vi "load channel file.vi"(8 "error in":errorcluster, 10 "Group Names":string[](array[string]), 11 "Channel List":path) -> (0 "error out":errorcluster, 1 "ACTIVE":T3 {"Channels in Group"."Card.Channel" format="%.2f"}, 2 "GROUP00":T3 {"Channels in Group"."Card.Channel" format="%.2f"}, 3 "Groups":T4(array[cluster]) {"Channels in Group"."Card.Channel" format="%.2f"}, 5 "Array":T1[](array[typedef]) {"Vfile (V)" format="%.1f V"; "Vswmax (V)" format="%#_g V"; "Iset (A)" format="%.2pA"; "Imon (A)" format="%.2pA"; "Vset (V)" format="%#_g V"; "Vmon (V)" format="%.1f V"})   [LabVIEW 2018]
uses:
  channel.ctl
  channel_cluster.ctl
  <vilib>/Utility/file.llb/Read Delimited Spreadsheet (string).vi
  string to bool small.vi
  fr string to dbl small.vi
  dec string to i32 small.vi
  CAEN globals.vi
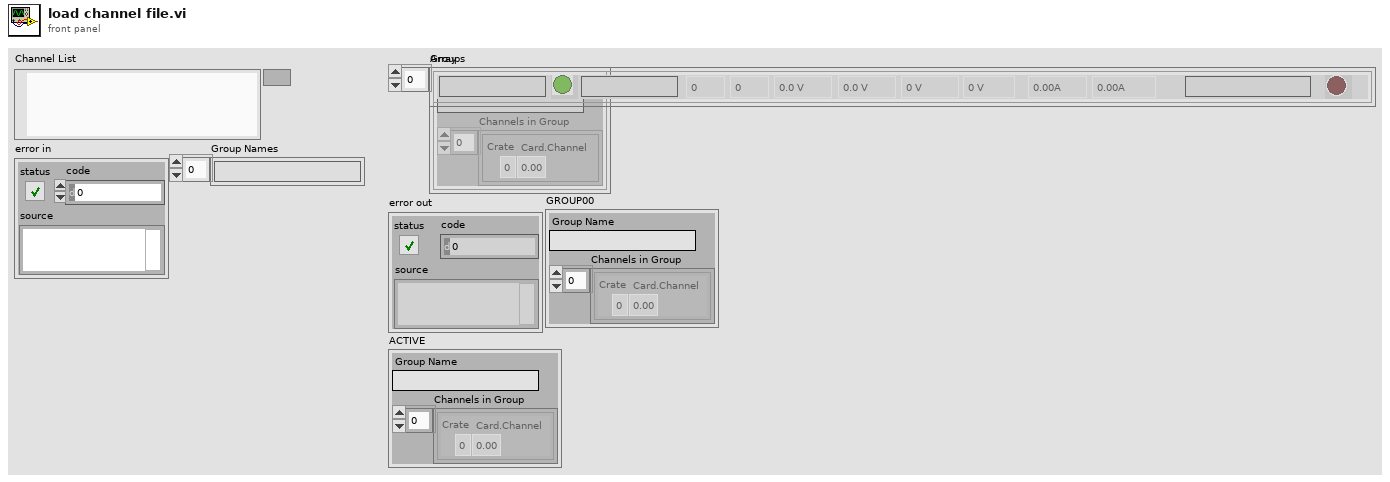
[diagram p1: front panel]
types:
  T1 = typedef "channel_cluster.ctl" = cluster{"Channel Name":string, "Crate":i32, "Card Type":string, "Card":i32, "Channel":i32, "Status Icon":picture, "Vmon (V)":dbl, "Vset (V)":dbl, "Imon (A)":dbl, "Iset (A)":dbl, "Timestamp":string, "ON/OFF":bool, "Status":string, "Vswmax (V)":dbl, "Flag":bool, "Vfile (V)":dbl, "Error Logged":bool[], "enable_file":bool}
  T2 = typedef "channel.ctl" = cluster{" Card.Channel":dbl, "Crate":i32}
  T3 = cluster{"Group Name":string, "Channels in Group":T2[]}
  T4 = cluster{"Group Name":string, "Channels in Group":T2[]}[]
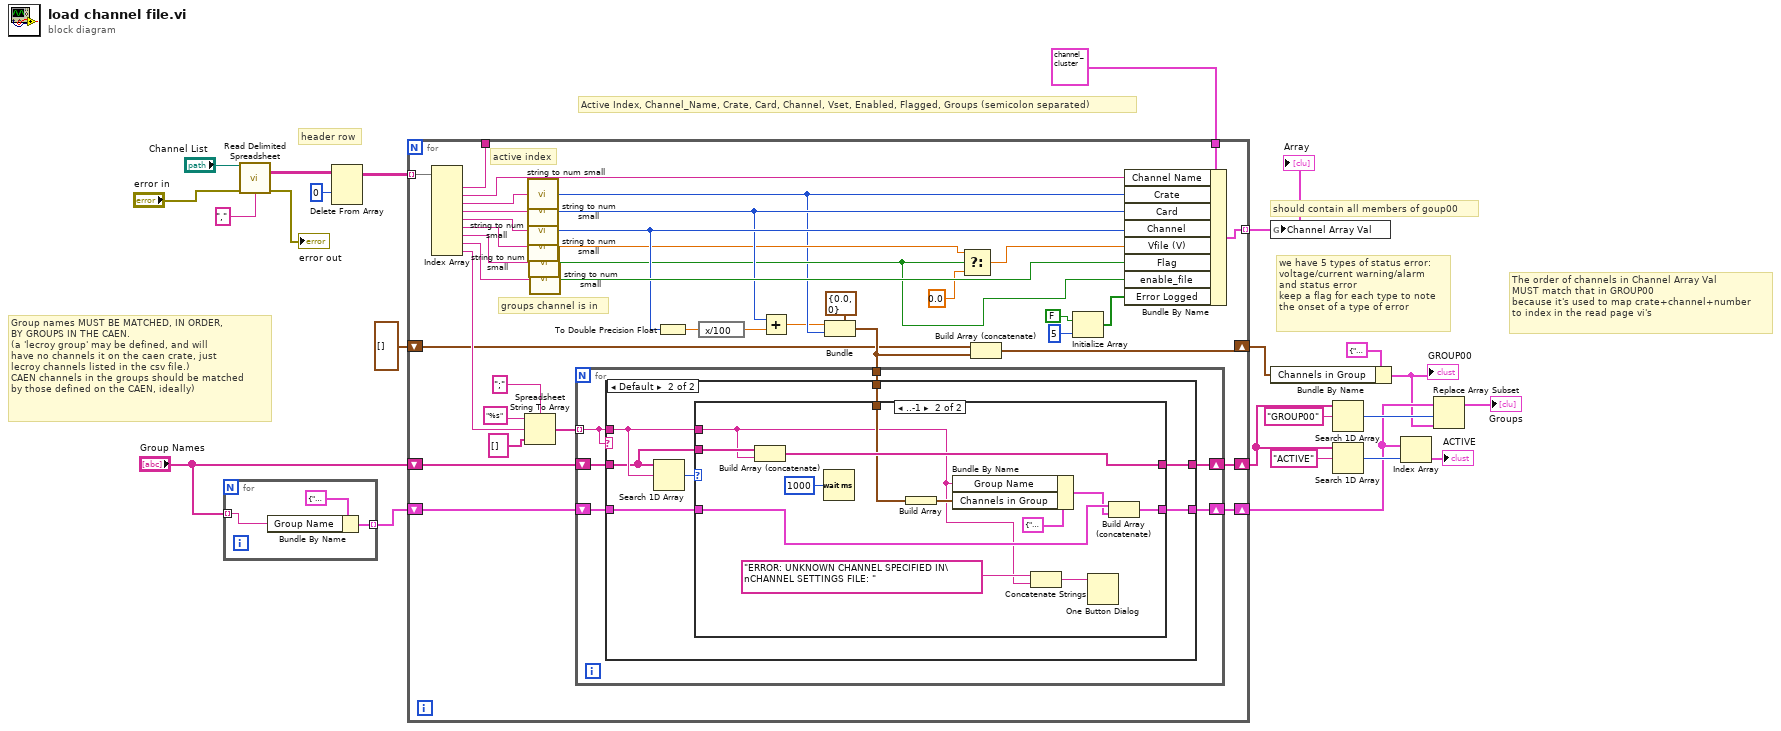
[diagram p0: block diagram]
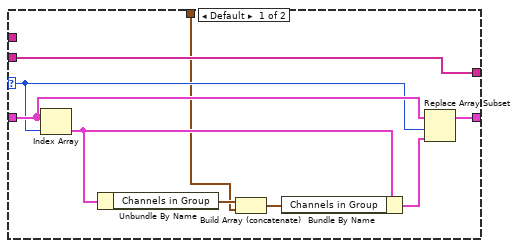
[diagram p3: hidden frame]
diagram:
  # "The order of channels in Channel Array Val\nMUST match that in GROUP00\nbecause it's used to map crate+channel+number\nto index in the read page vi's"
  # "Group names MUST BE MATCHED, IN ORDER,\nBY GROUPS IN THE CAEN. \n(a 'lecroy group' may be defined, and will\nhave no channels it on the caen crate, just\nlecroy channels listed in the csv file.)\nCAEN channels in the groups should be matched\nby those defined on the CAEN, ideally)"
  # "we have 5 types of status error:\nvoltage/current warning/alarm\nand status error\nkeep a flag for each type to note\nthe onset of a type of error"
  # "header row"
  # "should contain all members of goup00"
  # "Active Index, Channel_Name, Crate, Card, Channel, Vset, Enabled, Flagged, Groups (semicolon separated)"
  n1 = for {
    tunnel: "Group Names" -> [w26] mode=indexing
    tunnel: [w24] -> w1 mode=indexing
    n2 = Bundle By Name(cluster=T3 {"Group Name"="VETO", "Channels in Group"=[]}, "Group Name"=w26) -> (w24:T3)
  }
  n3 = call-poly <vilib>:"Read Delimited Spreadsheet.vi"("file path (dialog if empty)"="Channel List", "error in (no error)"="error in", "delimiter (\\t)"="," ("delimiter (\\t)")) -> ("all rows"=w11:string[][], "error out"=→"error out":errorcluster)  [unwired: 7 in, 4 out]
  n4 = Delete From Array(array=w11, index (row)=0) -> (array with subset deleted=w10:string[][])  [unwired: 2 in, 1 out]
  n5 = for {
    shift-right: [w46] -> w17
    shift-left: "Group Names" -> [w48]
    shift-right: [w45] -> w5
    shift-left: w1 -> [w47]
    tunnel: w10 -> [w64] mode=indexing
    tunnel: [w55] -> w21 mode=indexing
    tunnel: T1 {"Channel Name"="", "Crate"=0, "Card Type"="", "Card"=0, "Channel"=0, "Status Icon"=bytes[0], "Vmon (V)"=0.0, "Vset (V)"=0.0, "Imon (A)"=0.0, "Iset (A)"=0.0, "Timestamp"="", "ON/OFF"=FALSE, "Status"="", "Vswmax (V)"=0.0, "Flag"=FALSE, "Vfile (V)"=0.0, "Error Logged"=[], "enable_file"=FALSE} ("Channel cluster") -> [w51]
    tunnel: [w40] -> _
    shift-right: [w27] -> w6
    shift-left: T2[] [] -> [w28]
    # "groups channel is in"
    # "active index"
    n6 = Index Array(array=w64) -> (element #1=w40:string, element #2=w63:string, element #3=w62:string, element #4=w61:string, element #5=w60:string, element #6=w59:string, element #7=w58:string, element #8=w56:string, element #9=w54:string)  [unwired: 9 in]
    n7 = Spreadsheet String To Array(delimiter (Tab)=";", format string="%s" ("delimiter (Tab)"), spreadsheet string=w54, array type (2D Dbl)=string[] [] ("all rows")) -> (array=w49:string[])
    n8 = call-poly "string to num small.vi"("String"=w62) -> ("number"=w31:i32)  [unwired: 14 in]
    n9 = call-poly "string to num small.vi"("String"=w61) -> ("number"=w41:i32)  [unwired: 14 in]
    n10 = call-poly "string to num small.vi"("String"=w60) -> ("number"=w43:i32)  [unwired: 14 in]
    n11 = call-poly "string to num small.vi"("String"=w59) -> ("number"=w39:dbl)  [unwired: 14 in]
    n12 = call-poly "string to num small.vi"("String"=w58) -> ("number"=w33:bool)  [unwired: 14 in]
    n13 = call-poly "string to num small.vi"("String"=w56) -> ("number"=w57:bool)  [unwired: 14 in]
    n14 = To Double Precision Float(number=w43) -> (double precision float=w44:dbl)
    n15 = expression code="x/100"(w44) -> (w42:dbl)
    n16 = Add(x=w41, y=w42) -> (x+y=w30:dbl)
    n17 = Bundle(cluster=T2 {" Card.Channel"=0.0, "Crate"=0} ("Channel"), "Card.Channel"=w30, "Crate"=w31) -> (w29:T2)
    n18 = for {
      tunnel: w49 -> [w65] mode=indexing
      shift-right: [w69] -> w46
      shift-left: w48 -> [w70]
      shift-right: [w67] -> w45
      shift-left: w47 -> [w68]
      tunnel: w29 -> [w66]
      n19 = case shown="Default" w65 {
        tunnel: w65 -> [_ w79]
        tunnel: w70 -> [w72 w77]
        tunnel: [w72 w76] -> w69
        tunnel: w68 -> [w71 w75]
        tunnel: [w71 w74] -> w67
        tunnel: w66 -> [_ w73]
        frame "GROUP00" {
          # "ignore GROUP00; we'll make it external\n(means we don't need to rely on the user\nto have GROUP00 specified for every\nchannel in the table, or check for duplicates)"
        }
        frame Default {
          n20 = Search 1D Array(1D array=w77, element=w79) -> (index of element=w78:i32)  [unwired: 1 in]
          n21 = case shown="..-1" w78 {
            selector: w78 -> [w82 _]
            tunnel: w79 -> [_ w89]
            tunnel: w77 -> [w88 w100]
            tunnel: [w88 w99] -> w76
            tunnel: w75 -> [w87 w95]
            tunnel: [w86 w96] -> w74
            tunnel: w73 -> [w80 w93]
            frame Default {
              n22 = Index Array(array=w87, index=w82) -> (element=w84:T3)
              n23 = Unbundle By Name(w84) -> ("Channels in Group"=w85:T2[])
              n24 = Build Array (concatenate)(w85, w80) -> (w81:T2[])
              n25 = Bundle By Name(cluster=w84, "Channels in Group"=w81) -> (w83:T3)
              n26 = Replace Array Subset(array=w87, new element=w83, index=w82) -> (w86:T4)
            }
            frame ..-1 {
              n27 = Build Array (concatenate)(w100, w89) -> (w99:string[])
              n28 = Wait (ms)(milliseconds to wait=u32 1000) -> ()  [unwired: 1 out]
              n29 = Build Array(w93) -> (w97:T2[])
              n30 = Bundle By Name(cluster=T3 {"Group Name"="VETO", "Channels in Group"=[]}, "Group Name"=w89, "Channels in Group"=w97) -> (w94:T3)
              n31 = Concatenate Strings("ERROR: UNKNOWN CHANNEL SPECIFIED IN\nCHANNEL SETTINGS FILE: " ("message"), w89) -> (w91:string)
              n32 = One Button Dialog(message=w91) -> ()  [unwired: 1 in, 1 out]
              n33 = Build Array (concatenate)(w95, w94) -> (w96:T4)
            }
          }
        }
      }
    }
    n34 = Select(t=w39, s=w33, f=0.0) -> (s? t:f=w38:dbl)
    n35 = Build Array (concatenate)(w28, w29) -> (w27:T2[])
    n36 = Initialize Array(FALSE, 5 ("index (row)")) -> (w36:bool[])
    n37 = Bundle By Name(cluster=w51, "Channel Name"=w63, "Crate"=w31, "Card"=w41, "Channel"=w43, "Vfile (V)"=w38, "Flag"=w57, "enable_file"=w33, "Error Logged"=w36) -> (w55:T1)
  }
  "Array" <- w21
  n38 = global write "CAEN globals.vi" "Channel Array Val"(w21) -> ()
  n39 = Bundle By Name(cluster=T3 {"Group Name"="GROUP00", "Channels in Group"=[]}, "Channels in Group"=w6) -> (w3:T3)
  "GROUP00" <- w3
  n40 = Search 1D Array(1D array=w17, element="GROUP00") -> (index of element=w14:i32)  [unwired: 1 in]
  n41 = Search 1D Array(1D array=w17, element="ACTIVE") -> (index of element=w13:i32)  [unwired: 1 in]
  n42 = Index Array(array=w5, index=w13) -> (element=→"ACTIVE":T3)
  n43 = Replace Array Subset(array=w5, new element=w3, index=w14) -> (→"Groups":T4)
